vi "Sound Warning.vi"(8 "error in (no error)":errorcluster, 11 "Electric Fence in":refnum<class "Electric Fence.lvclass">) -> (0 "error out":errorcluster, 3 "Electric Fence out":refnum<class "Electric Fence.lvclass">)   [LabVIEW 2014, in "Electric Fence.lvclass"]
uses:
  Electric Fence.lvclass
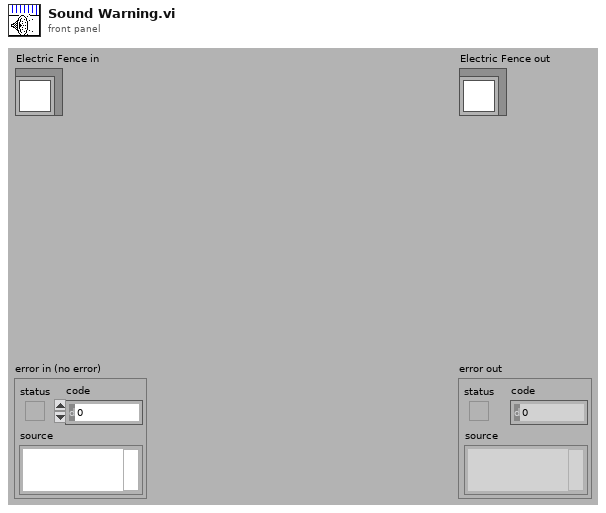
[diagram p1: front panel]
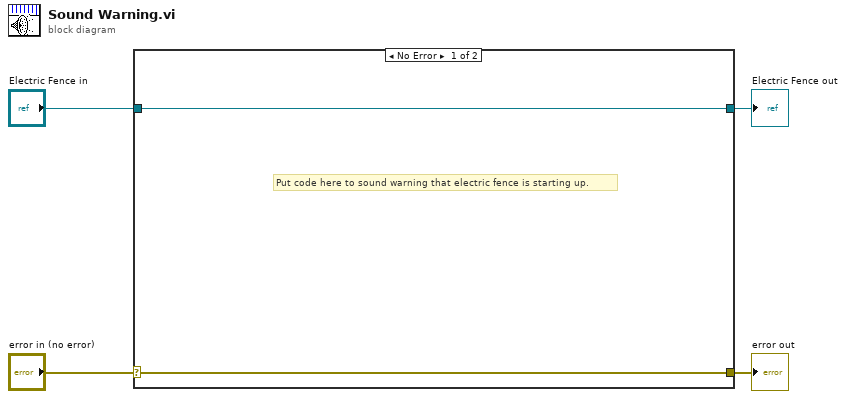
[diagram p0: block diagram]
diagram:
  n1 = case shown="No Error" "error in (no error)" {
    selector: "error in (no error)" -> [w5 w8]
    tunnel: [w5 w8] -> w3
    tunnel: [w6 w7] -> w1
    tunnel: "Electric Fence in" -> [w6 w7]
    frame No Error {
      # "Put code here to sound warning that electric fence is starting up."
    }
    frame Error {
    }
  }
  "error out" <- w3
  "Electric Fence out" <- w1
